vi "Asylum_GetDevices.vi"(8 "error in (no error)":errorcluster, 11 "Application":refnum<k7>) -> (0 "error out":errorcluster, 2 "Devices":string, 3 "Application":refnum<k7>)   [LabVIEW 2020]
doc: "Returns a list of all devices currently connected in the MFP-3D system. Please note that this returns the results from the last scan. If devices have been unplugged since the last scan, the results of this function will be inaccurate. You probably want to call td_ScanForDevices before using this function.\n\nParameters\n\nwave A text wave in which you want to store the devices. The row label contains the name of the device as it is known on the bus and the string value contains the type of the device. These two are often the same unless you have multiple devices of the same type on the bus.\n\nFunction Result\n\nSee MFP-3D Controller Error Code Reference\n\nSee Also td_ScanForDevices"
panel:
  in  "textWave":string="textWave"
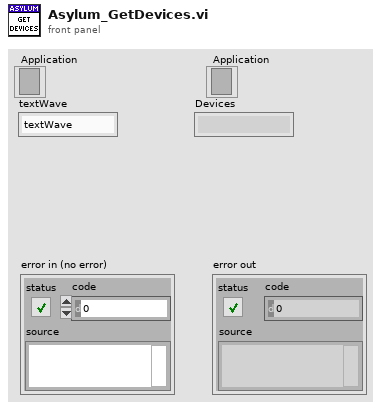
[diagram p1: front panel]
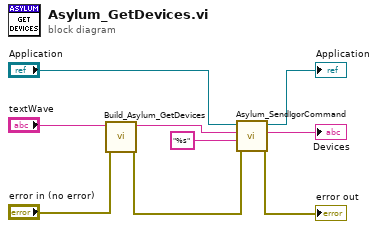
[diagram p0: block diagram]
diagram:
  n1 = call "Build_Asylum_GetDevices.vi"("error in (no error)"="error in (no error)", "textWave"="textWave") -> ("error out"=w9:errorcluster, "Command"=w7:string)  [unwired: 8 in]
  n2 = call "Asylum_SendIgorCommand.vi"("error in (no error)"=w9, "Format"="%s", "command"=w7, "Application In"="Application") -> ("error out"=→"error out":errorcluster, "results"=→"Devices":string, "Application Out"=→"Application":refnum<k7>)  [unwired: 4 in, 1 out]
